vi "CreatePizza.vi"(8 "error in (no error)":errorcluster, 11 "ChicagoPizzaStore in":refnum<class "NYPizzaStore.lvclass">) -> (0 "error out":errorcluster, 2 "YourPizzay":string, 3 "ChicagoPizzaStore out":refnum<class "NYPizzaStore.lvclass">)   [LabVIEW 2013, in "NYPizzaStore.lvclass"]
uses:
  NYPizzaStore.lvclass
  NYPizzaIngredientFactory.lvclass/NYPizzaIngredientFactory.lvclass
panel:
  # "我是紐約的比薩店"
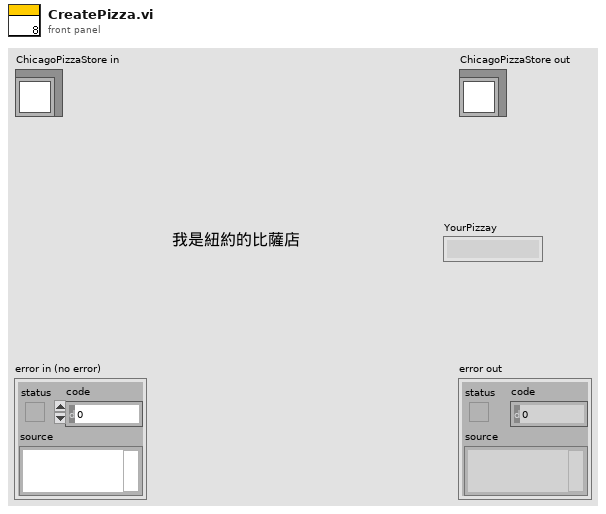
[diagram p1: front panel]
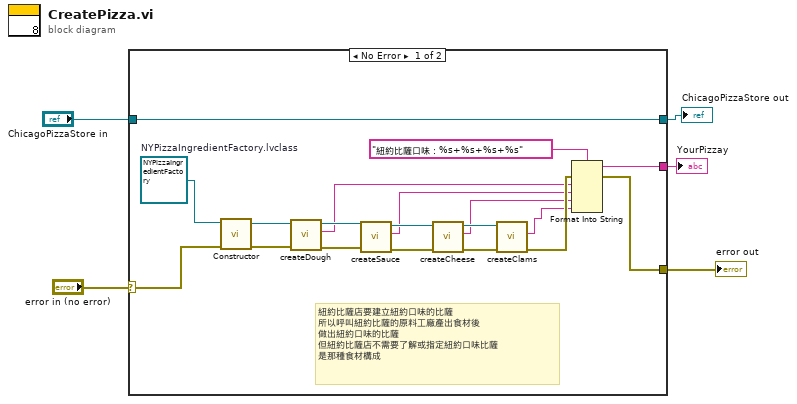
[diagram p0: block diagram]
diagram:
  n1 = case shown="No Error" "error in (no error)" {
    selector: "error in (no error)" -> [w16 w25]
    tunnel: [w15 w26] -> w4
    tunnel: "ChicagoPizzaStore in" -> [w15 w26]
    tunnel: [w7 w25] -> w2
    tunnel: [w6 _] -> w1
    frame No Error {
      w14 = refnum<class "NYPizzaIngredientFactory.lvclass"> refnum  # NYPizzaIngredientFactory.lvclass
      # "紐約比薩店要建立紐約口味的比薩\n所以呼叫紐約比薩的原料工廠產出食材後\n做出紐約口味的比薩\n但紐約比薩店不需要了解或指定紐約口味比薩\n是那種食材構成"
      n2 = call-dynamic "Constructor.vi"("error in (no error)"=w16, "NYPizzaIngredientFactory in"=w14) -> ("error out"=w20:errorcluster, "NYPizzaIngredientFactory out"=w24:refnum<class "NYPizzaIngredientFactory.lvclass">)  [unwired: 8 in]
      n3 = call-dynamic "createDough.vi"("error in (no error)"=w20, "NYPizzaIngredientFactory in"=w24) -> ("error out"=w19:errorcluster, "Ingredients"=w11:string, "NYPizzaIngredientFactory out"=w23:refnum<class "NYPizzaIngredientFactory.lvclass">)  [unwired: 7 in]
      n4 = call-dynamic "createSauce.vi"("error in (no error)"=w19, "NYPizzaIngredientFactory in"=w23) -> ("error out"=w18:errorcluster, "Ingredients"=w10:string, "NYPizzaIngredientFactory out"=w22:refnum<class "NYPizzaIngredientFactory.lvclass">)  [unwired: 7 in]
      n5 = call-dynamic "createCheese.vi"("error in (no error)"=w18, "NYPizzaIngredientFactory in"=w22) -> ("error out"=w17:errorcluster, "Ingredients"=w9:string, "NYPizzaIngredientFactory out"=w21:refnum<class "NYPizzaIngredientFactory.lvclass">)  [unwired: 7 in]
      n6 = call-dynamic "createClams.vi"("error in (no error)"=w17, "NYPizzaIngredientFactory in"=w21) -> ("error out"=w12:errorcluster, "Ingredients"=w8:string)  [unwired: 7 in, 1 out]
      n7 = Format Into String(format string="紐約比薩口味：%s+%s+%s+%s", error in=w12, w11, w10, w9, w8) -> (resulting string=w6:string, error out=w7:errorcluster)  [unwired: 1 in]
    }
    frame Error {
    }
  }
  "error out" <- w2
  "ChicagoPizzaStore out" <- w4
  "YourPizzay" <- w1
